vi "Task6.vi"(11 "Button":bool[](array[boolean])) -> (3 "Numeric":u32)   [LabVIEW 2017]
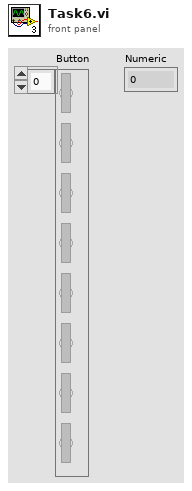
[diagram p1: front panel]
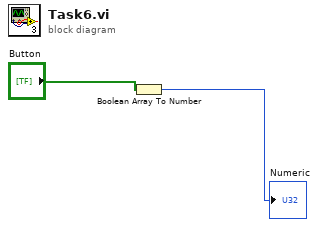
[diagram p0: block diagram]
diagram:
  n1 = Boolean Array To Number(Boolean array="Button") -> (number=→"Numeric":u32)
